vi "Main.vi"(8 "error in":errorcluster caption="entrée d'erreur") -> (0 "error out":errorcluster caption="sortie d'erreur")   [LabVIEW 2026]
uses:
  APE codes/LabVIEW/LV13/Basic Example/cluster/tcp client action.ctl
panel:
  out "Sent string":string
  out "Answer":string
  in  "Host":string="127.0.0.1"
  in  "Port":u16=51019
  in  "Value":dbl
  in  "Command":T1(ring)
  in  "Quit":bool
  in  "Send":bool
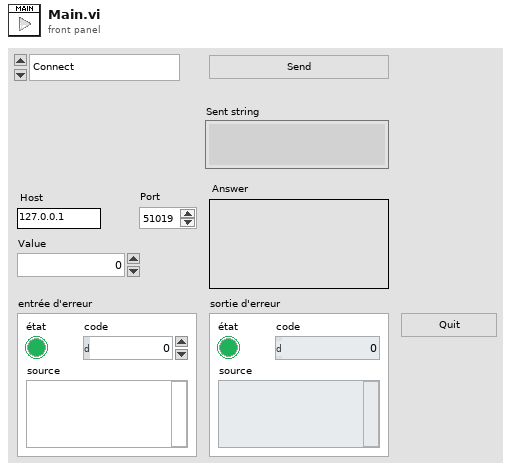
[diagram p1: front panel]
types:
  T1 = enum16{"Connect", "Disconnet", "set_wavelength", "set_signal_power", "set_ir_power", "set_delay", "set_signal_shutter", "set_ir_shutter", "set_main_shutter", "parameters?"}
  T2 = typedef "tcp client action.ctl" = enum16{"Connect", "Write", "Query", "Disconnect"}
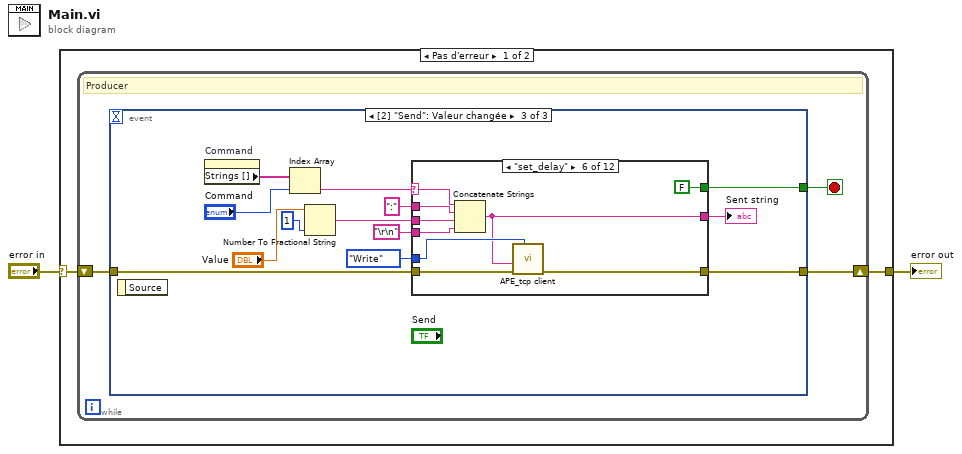
[diagram p0: block diagram]
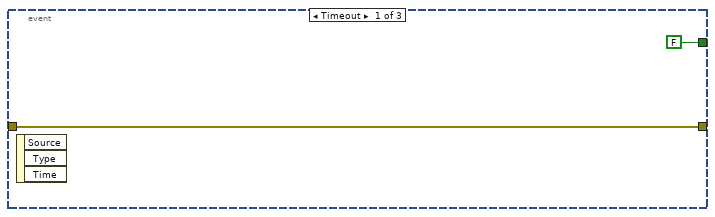
[diagram p2: hidden frame]
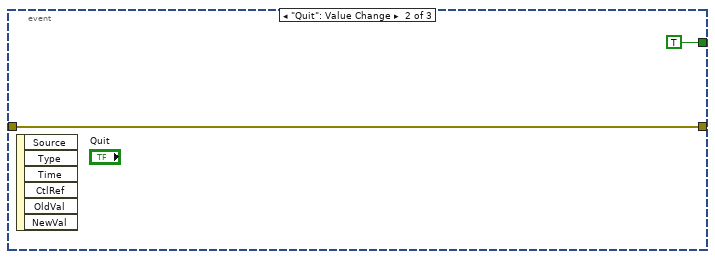
[diagram p3: hidden frame]
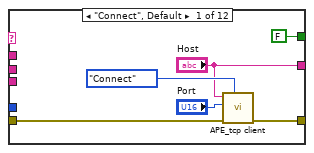
[diagram p4: hidden frame]
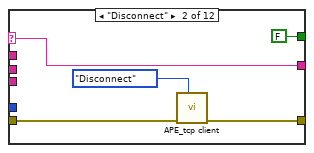
[diagram p5: hidden frame]
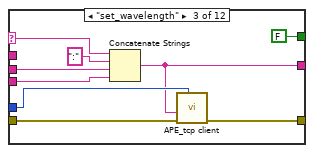
[diagram p6: hidden frame]
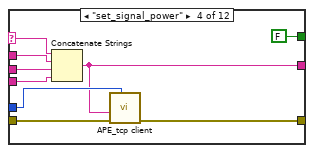
[diagram p7: hidden frame]
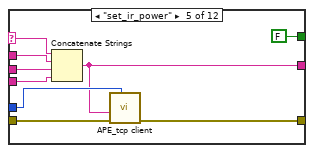
[diagram p8: hidden frame]
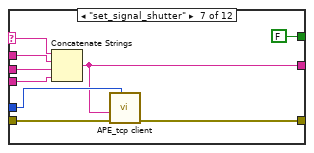
[diagram p9: hidden frame]
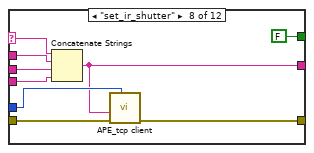
[diagram p10: hidden frame]
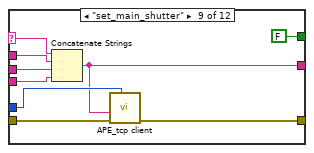
[diagram p11: hidden frame]
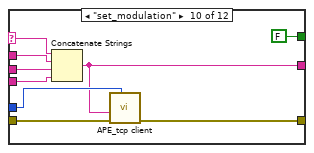
[diagram p12: hidden frame]
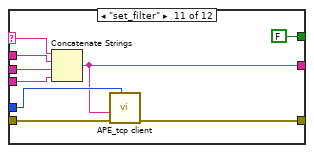
[diagram p13: hidden frame]
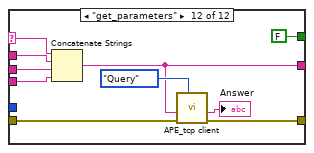
[diagram p14: hidden frame]
diagram:
  n1 = case shown="Pas d'erreur" "error in" {
    selector: "error in" -> [w4 w127]
    tunnel: [w3 w127] -> w1
    frame No Error {
      n2 = while {
        shift-right: [w6] -> w3
        shift-left: w4 -> [w7]
        stop <- w5 stop-if-true
        # "Producer"
        n3 = event shown="[2] \"Send\": Valeur changée" {
          selector: _ -> [_ _ _]
          dyn-events: _ -> [_ _ _]
          timeout: _ -> [_ _ _]
          tunnel: w7 -> [w9 w11 w21]
          tunnel: [w9 w11 w20] -> w6
          tunnel: [FALSE TRUE w14] -> w5
          event Timeout {
            n4 = event-data() -> ()  [unwired: 1 in, 3 out]
          }
          event "Quit": Value Change {
            n5 = event-data() -> ()  [unwired: 1 in, 6 out]
          }
          event "Send": Value Change {
            n6 = event-data() -> ()  [unwired: 1 in, 1 out]
            n7 = property on="Command" class="Énum (strict)"() -> ("Strings []"=w24:string[])  [unwired: 2 in, 2 out]
            n8 = Index Array(array=w24, index="Command") -> (element=w22:string)
            n9 = Number To Fractional String(number="Value", precision (6)=i16 1 ("précision (6)")) -> (F-format string=w17:string)  [unwired: 2 in]
            n10 = case shown="\"set_delay\"" w22 {
              selector: w22 -> [_ w31 w40 w50 w59 w68 w77 w86 w95 w104 w113 w123]
              tunnel: w21 -> [w28 w35 w42 w52 w61 w70 w79 w88 w97 w106 w115 w125]
              tunnel: [w27 w34 w41 w51 w60 w69 w78 w87 w96 w105 w114 w124] -> w20
              tunnel: w17 -> [_ _ w43 w53 w62 w71 w80 w89 w98 w107 w116 w126]
              tunnel: "\r\n" -> [_ _ w36 w49 w57 w66 w76 w84 w93 w102 w111 w120]
              tunnel: ":" ("chaîne") -> [_ _ _ w48 w58 w67 w75 w85 w94 w101 w112 w121]
              tunnel: [FALSE FALSE FALSE FALSE FALSE FALSE FALSE FALSE FALSE FALSE FALSE FALSE] -> w14
              tunnel: tcp_client_action."Write" ("Action") -> [_ _ w39 w47 w56 w65 w74 w82 w91 w100 w109 _]
              tunnel: ["Host" w31 w37 w45 w54 w63 w72 w81 w90 w99 w108 w117] -> w12
              frame "Connect", Default {
                n11 = call "APE_tcp client.vi"("Action"=tcp_client_action."Connect", "error in"=w28, "TCP Port"="Port", "Host"="Host") -> ("error out"=w27:errorcluster)  [unwired: 6 in, 1 out]
              }
              frame "Disconnect" {
                n12 = call "APE_tcp client.vi"("Action"=tcp_client_action."Disconnect", "error in"=w35) -> ("error out"=w34:errorcluster)  [unwired: 8 in, 1 out]
              }
              frame "set_wavelength" {
                n13 = Concatenate Strings(w40, ":" ("chaîne"), w43, w36) -> (w37:string)
                n14 = call "APE_tcp client.vi"("Action"=w39, "error in"=w42, "Command"=w37) -> ("error out"=w41:errorcluster)  [unwired: 7 in, 1 out]
              }
              frame "set_signal_power" {
                n15 = Concatenate Strings(w50, w48, w53, w49) -> (w45:string)
                n16 = call "APE_tcp client.vi"("Action"=w47, "error in"=w52, "Command"=w45) -> ("error out"=w51:errorcluster)  [unwired: 7 in, 1 out]
              }
              frame "set_ir_power" {
                n17 = Concatenate Strings(w59, w58, w62, w57) -> (w54:string)
                n18 = call "APE_tcp client.vi"("Action"=w56, "error in"=w61, "Command"=w54) -> ("error out"=w60:errorcluster)  [unwired: 7 in, 1 out]
              }
              frame "set_delay" {
                n19 = Concatenate Strings(w68, w67, w71, w66) -> (w63:string)
                n20 = call "APE_tcp client.vi"("Action"=w65, "error in"=w70, "Command"=w63) -> ("error out"=w69:errorcluster)  [unwired: 7 in, 1 out]
              }
              frame "set_signal_shutter" {
                n21 = Concatenate Strings(w77, w75, w80, w76) -> (w72:string)
                n22 = call "APE_tcp client.vi"("Action"=w74, "error in"=w79, "Command"=w72) -> ("error out"=w78:errorcluster)  [unwired: 7 in, 1 out]
              }
              frame "set_ir_shutter" {
                n23 = Concatenate Strings(w86, w85, w89, w84) -> (w81:string)
                n24 = call "APE_tcp client.vi"("Action"=w82, "error in"=w88, "Command"=w81) -> ("error out"=w87:errorcluster)  [unwired: 7 in, 1 out]
              }
              frame "set_main_shutter" {
                n25 = Concatenate Strings(w95, w94, w98, w93) -> (w90:string)
                n26 = call "APE_tcp client.vi"("Action"=w91, "error in"=w97, "Command"=w90) -> ("error out"=w96:errorcluster)  [unwired: 7 in, 1 out]
              }
              frame "set_modulation" {
                n27 = Concatenate Strings(w104, w101, w107, w102) -> (w99:string)
                n28 = call "APE_tcp client.vi"("Action"=w100, "error in"=w106, "Command"=w99) -> ("error out"=w105:errorcluster)  [unwired: 7 in, 1 out]
              }
              frame "set_filter" {
                n29 = Concatenate Strings(w113, w112, w116, w111) -> (w108:string)
                n30 = call "APE_tcp client.vi"("Action"=w109, "error in"=w115, "Command"=w108) -> ("error out"=w114:errorcluster)  [unwired: 7 in, 1 out]
              }
              frame "get_parameters" {
                n31 = Concatenate Strings(w123, w121, w126, w120) -> (w117:string)
                n32 = call "APE_tcp client.vi"("Action"=tcp_client_action."Query", "error in"=w125, "Command"=w117) -> ("error out"=w124:errorcluster, "Answer"=→"Answer":string)  [unwired: 7 in]
              }
            }
            "Sent string" <- w12
          }
        }
      }
    }
    frame Error {
    }
  }
  "error out" <- w1
